vi "CSTK_Icon_Creator_CreateLogo_ColorToLogo.vi"(4 "Double Click":bool, 6 "Button":u16, 7 "ArrayIndex":T1, 8 "错误输入（无错误）":errorcluster, 9 "右键单击颜色":u32, 10 "左键单击颜色":u32, 11 "LOGO输入":refnum<vi>) -> (0 "错误输出":errorcluster, 3 "LOGO输出":refnum<vi>)   [LabVIEW 2015, in "CSTK_Icon Creator.lvlib"]
uses:
  CSTK_Icon Creator.lvlib
  <vilib>/Utility/miscctls.llb/LVPoint32TypeDef.ctl
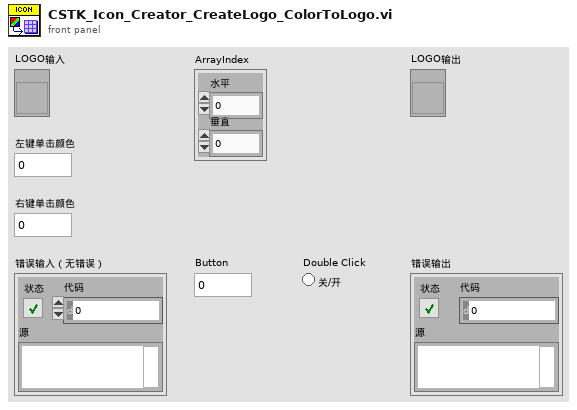
[diagram p1: front panel]
types:
  T1 = typedef "LVPoint32TypeDef.ctl" = cluster{"Horizontal":i32, "Vertical":i32}
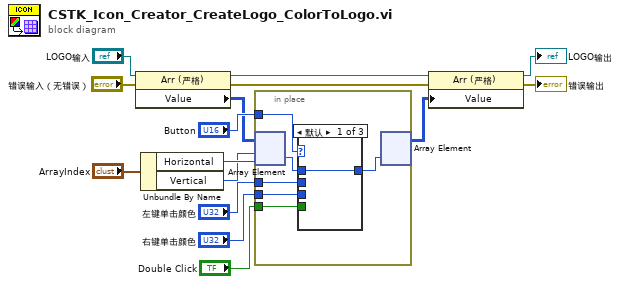
[diagram p0: block diagram]
diagram:
  n1 = property on="属性节点" class="Arr (严格)"(reference="LOGO输入", error in="错误输入（无错误）") -> (reference out=w2:refnum<vi>, error out=w9:errorcluster, "Value"=w7:u32[][])
  n2 = Unbundle By Name("ArrayIndex") -> ("Horizontal"=w11:i32, "Vertical"=w10:i32)
  n3 = in-place {
    in-place-border: "Button" -> [w21]
    in-place-border: "Double Click" -> [w18]
    in-place-border: "左键单击颜色" -> [w17]
    in-place-border: "右键单击颜色" -> [w16]
    n4 = in-place-array #1(w7, w10, w11) -> (w20:u32)
    n5 = case shown="默认" w21 {
      tunnel: [w22 w23 w24] -> w19
      tunnel: w20 -> [w22 _ _]
      tunnel: w18 -> [_ _ _]
      tunnel: w17 -> [_ w23 _]
      tunnel: w16 -> [_ _ w24]
      frame Default {
      }
      frame 1 {
      }
      frame 2 {
      }
    }
    n6 = in-place-array #1(w19) -> (w8:u32[][])  [unwired: 2 out]
  }
  n7 = property on="属性节点" class="Arr (严格)"(reference=w2, error in=w9, "Value"=w8) -> (reference out=→"LOGO输出":refnum<vi>, error out=→"错误输出":errorcluster)
